vi "Get SMO Public API.vi"(8 "error in (no error)":errorcluster, 11 "Inst.FP in":refnum<class "Inst.FP.lvclass">) -> (0 "error out":errorcluster, 2 "Commands":string[](array[string]), 3 "Inst.FP out":refnum<class "Inst.FP.lvclass">)   [LabVIEW 2019, in "Inst.FP.lvclass"]
uses:
  Inst.FP.lvclass
  C:/Program Files (x86)/National Instruments/LabVIEW 2019/user.lib/LevyLab/Instrument Framework/Instrument/Instrument.lvclass
  Typedefs/Inst.FP.Commands--Enum.ctl
  ae41134a-25c1-4b9b-a201-0c4851d23a24.vi
  <vilib>/Utility/Data Type/Get Type Information.vi
  <vilib>/Utility/Data Type/Get Numeric Information.vi
  <userlib>/_OpenG.lib/lvdata/lvdata.llb/Unwrap VVariant__ogtk.vi
  <userlib>/LevyLab/Instrument Framework/Instrument Types/Cryostat/Instrument.Cryostat.lvclass
  <userlib>/LevyLab/Instrument Framework/Instrument/Instrument.lvclass
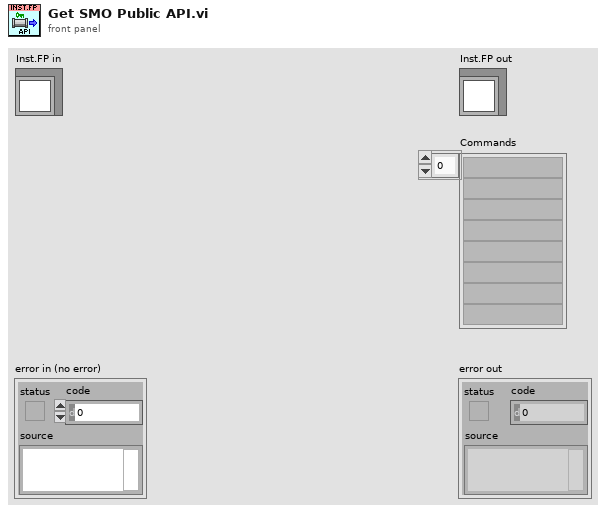
[diagram p1: front panel]
types:
  T1 = typedef "Inst.FP.lvclass/Inst.FP.Commands--Enum.ctl" = enum16{"getMode", "setMode", "pushButton"}
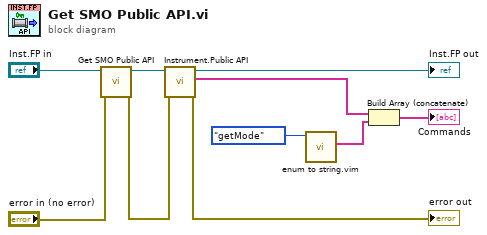
[diagram p0: block diagram]
diagram:
  n1 = call-parent "Get SMO Public API.vi"("error in (no error)"="error in (no error)", "Instrument.Cryostat in"="Inst.FP in") -> ("error out"=w4:errorcluster, "Instrument.Cryostat out"=w2:refnum<class "Inst.FP.lvclass">)  [unwired: 7 in, 1 out]
  n2 = call <userlib>:"Instrument.Public API.vi"("error in (no error)"=w4, "Instrument in"=w2) -> ("error out"=→"error out":errorcluster, "commands (this level)"=w5:string[], "Instrument out"=→"Inst.FP out":refnum<class "Inst.FP.lvclass">)  [unwired: 7 in]
  n3 = call "enum to string.vim"("enum in"=Inst.FP.Commands--Enum."getMode" ("Commands")) -> ("strings out"=w6:string[])  [unwired: 9 in, 1 out]
  n4 = Build Array (concatenate)(w5, w6) -> (→"Commands":string[])
